vi "Write Active.vi"(8 "error in (no error)":errorcluster, 10 "Active":bool, 11 "Button in":refnum<class "Button.lvclass">) -> (0 "error out":errorcluster, 3 "Button out":refnum<class "Button.lvclass">)   [LabVIEW 2019, in "Button.lvclass"]
uses:
  Button.lvclass
  Button.lvclass/Button.ctl
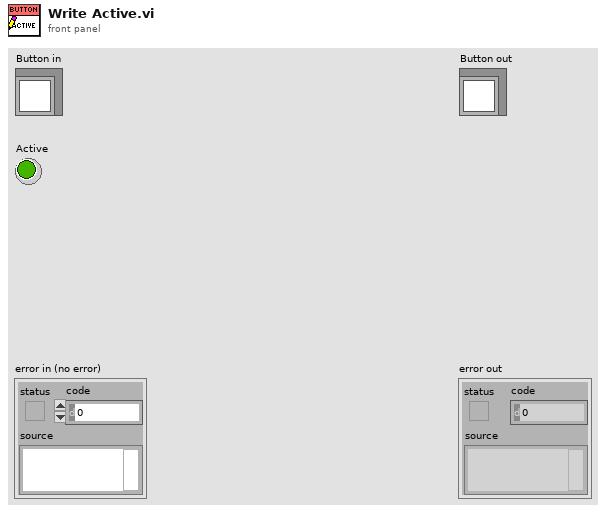
[diagram p1: front panel]
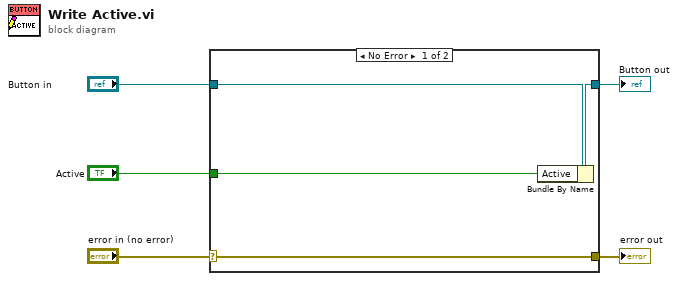
[diagram p0: block diagram]
diagram:
  n1 = case shown="No Error" "error in (no error)" {
    selector: "error in (no error)" -> [w9 w10]
    tunnel: [w9 w10] -> w4
    tunnel: [w7 w11] -> w2
    tunnel: "Button in" -> [w8 w11]
    tunnel: "Active" -> [w6 _]
    frame No Error {
      n2 = Bundle By Name(cluster=w8, "Active"=w6) -> (w7:refnum<class "Button.lvclass">)
    }
    frame Error {
    }
  }
  "error out" <- w4
  "Button out" <- w2
